vi "Get Config Path.vi"(8 "error in (no error)":errorcluster, 11 "gScript Interpreter in":refnum<class "gScript Interpreter.lvclass">) -> (0 "error out":errorcluster, 2 "INI Config Path":path, 3 "gScript Interpreter out":refnum<class "gScript Interpreter.lvclass">)   [LabVIEW 2023, in "gScript Interpreter.lvclass"]
uses:
  gScript Interpreter.lvclass
  <vilib>/Utility/sysdir.llb/System Directory Type.ctl
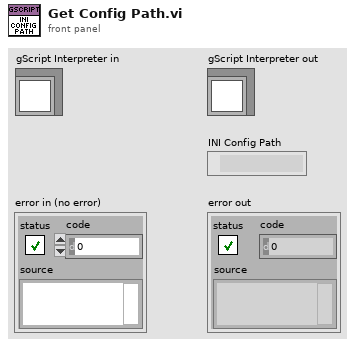
[diagram p1: front panel]
types:
  T1 = typedef "System Directory Type.ctl" = i32
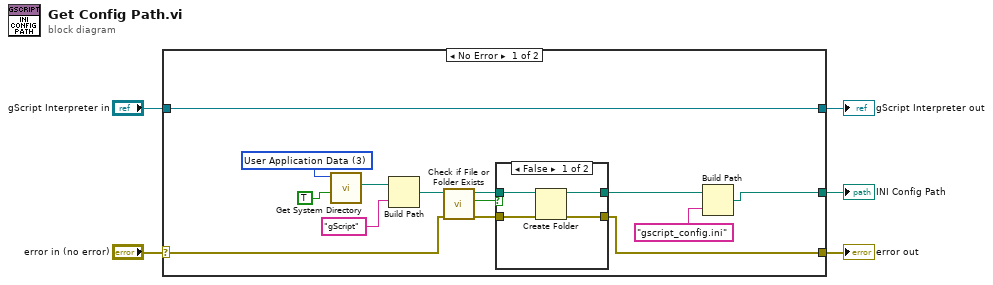
[diagram p0: block diagram]
diagram:
  n1 = case shown="No Error" "error in (no error)" {
    selector: "error in (no error)" -> [w10 w27]
    tunnel: [w9 w27] -> w4
    tunnel: [w19 w26] -> w2
    tunnel: "gScript Interpreter in" -> [w19 w26]
    tunnel: [w6 _] -> w1
    frame No Error {
      w17 = T1 3 items=["User Home"=0, "User Desktop"=1, "User Documents"=2, "User Application Data"=3, "User Preferences"=4, "User Temporary"=5, "Public Documents"=6, "Public Application Data"=7, "Public Preferences"=8, "Public Cache"=13, "System Core Libraries"=9, "System Installed Libraries"=10, "Application Files"=11, "Boot Volume Root"=12] ("system directory type")
      n2 = call <vilib>:"Get System Directory.vi"("create directory if not found? (F)"=TRUE, "system directory type"=w17) -> ("system directory"=w16:path)  [unwired: 9 in]
      n3 = Build Path(base path=w16, name or relative path="gScript") -> (appended path=w14:path)
      n4 = call <vilib>:"Check if File or Folder Exists.vi"("error in (no error)"=w10, "path"=w14) -> ("error out"=w12:errorcluster, "file or folder exists?"=w13:bool, "dup path"=w11:path)  [unwired: 7 in]
      n5 = case shown="False" w13 {
        tunnel: w12 -> [w23 w24]
        tunnel: w11 -> [w22 w25]
        tunnel: [w21 w24] -> w9
        tunnel: [w20 w25] -> w7
        frame False {
          n6 = Create Folder(path (use dialog)=w22, error in=w23) -> (created path=w20:path, error out=w21:errorcluster)  [unwired: 1 in, 1 out]
        }
        frame True {
        }
      }
      n7 = Build Path(base path=w7, name or relative path="gscript_config.ini") -> (appended path=w6:path)
    }
    frame Error {
    }
  }
  "error out" <- w4
  "gScript Interpreter out" <- w2
  "INI Config Path" <- w1
